vi "GPIOs.vi"(8 "error in (no error)":errorcluster, 11 "SPI in":refnum<class "SPI.lvclass">) -> (0 "error out":errorcluster, 1 "RX GPIO":T1, 2 "TX GPIO":T1, 3 "SPI out":refnum<class "SPI.lvclass">, 4 "SCK GPIO":T1)   [LabVIEW 2024, in "CTI.lvlib" / "SPI.lvclass"]
uses:
  SPI.lvclass
  GPIO Number.ctl
  SPI.lvclass/SPI.ctl
  CTI.lvlib
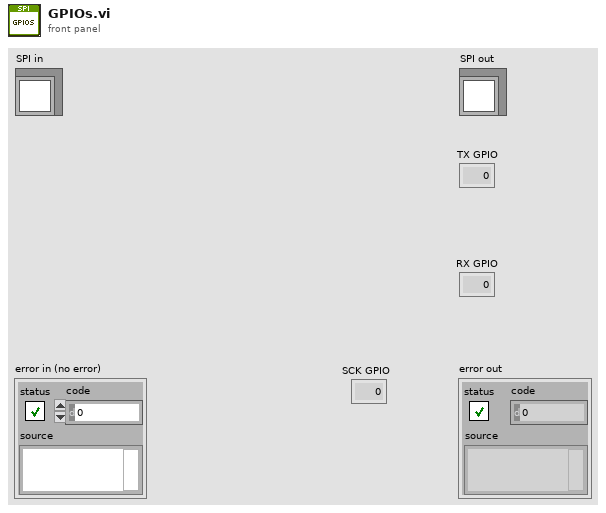
[diagram p1: front panel]
types:
  T1 = typedef "CTI.lvlib/GPIO Number.ctl" = i8
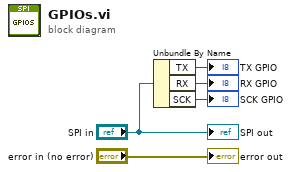
[diagram p0: block diagram]
diagram:
  n1 = Unbundle By Name("SPI in") -> ("TX"=→"TX GPIO":T1, "RX"=→"RX GPIO":T1, "SCK"=→"SCK GPIO":T1)
  "error out" <- "error in (no error)"
  "SPI out" <- "SPI in"
